vi "Log Line.vi"(7 "average exponent":i32=4, 8 "current time":timestamp, 9 "firmware revision":string(combo), 10 "units":i32(ring)=1 items=["NS"=1, "DS"=2, "KO"=3, "GO"=4, "JP"=5], 11 "measurement results":T1) -> (2 "log line":string caption="Result")   [LabVIEW 2019, in "Andeen-Hagerling 2700A.lvlib"]
doc: "Create a text line based on measurement parameters that can be used to create a measurement log file."
uses:
  Andeen-Hagerling 2700A.lvlib
  Instance           1 16Saved   Log Line .vi
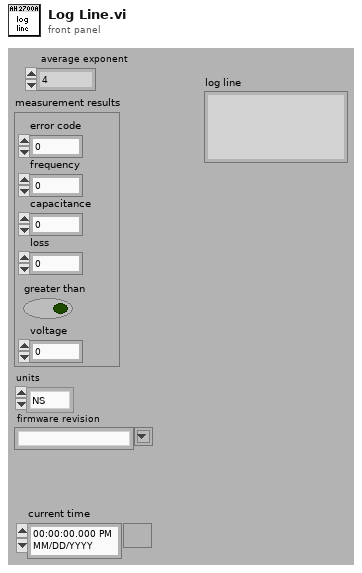
[diagram p1: front panel]
types:
  T1 = cluster{"error code":i32, "frequency":dbl, "capacitance":dbl, "loss":dbl, "greater than":bool, "voltage":dbl}
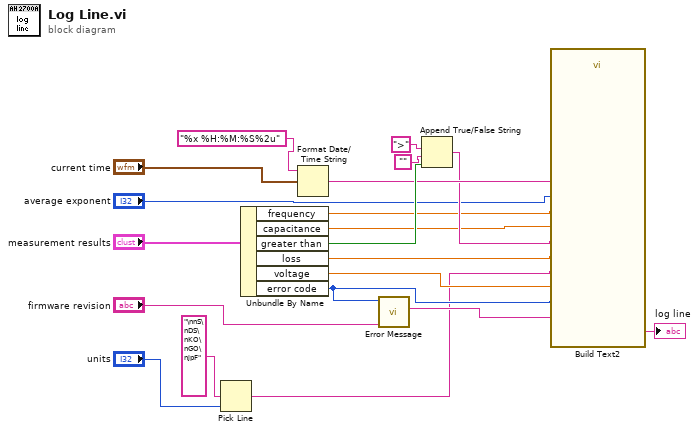
[diagram p0: block diagram]
diagram:
  n1 = Pick Line(multi-line string="\nnS\nDS\nKO\nGO\njpF", line index="units") -> (output string=w7:string)  [unwired: 1 in]
  n2 = Unbundle By Name("measurement results") -> ("frequency"=w3:dbl, "capacitance"=w4:dbl, "greater than"=w17:bool, "loss"=w6:dbl, "voltage"=w8:dbl, "error code"=w9:i32)
  n3 = Format Date/Time String(time format string (%c)="%x %H:%M:%S%2u", seconds (now)="current time") -> (date/time string=w11:string)  [unwired: 1 in]
  n4 = call "Error Message.vi"("firmware revision"="firmware revision", "error number"=w9) -> ("error message"=w10:string)  [unwired: 9 in]
  n5 = Append True/False String(1:w17, 2:"", 3:">" ("true string")) -> (0:w5:string)  [unwired: 1 in]
  n6 = call "Build Text2"("time"=w11, "average exponent"="average exponent", "frequency"=w3, "capacitance"=w4, "greater than"=w5, "loss"=w6, "units"=w7, "voltage"=w8, "error code"=w9, "error message"=w10) -> ("Result"=→"log line":string)  [unwired: 16 in, 1 out]
